vi "OceanOpticsInitialize.vi"(8 "error in (no error)":errorcluster, 11 "Numeric":i32) -> (0 "error out":errorcluster, 1 "getName":string, 2 "getSerialNumber":string, 3 ".NET Refnum out":refnum<k24>)   [LabVIEW 2016]
uses:
  C:/Program Files (x86)/Ocean Optics/OmniDriver/OOI_HOME/NETOmniDriver-NET40.dll
  Program Files (x86)/Ocean Optics/OmniDriver/OOI_HOME/NETOmniDriver-NET40.dll
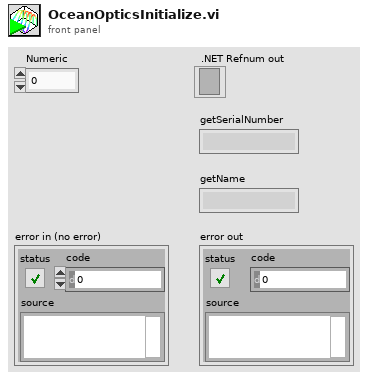
[diagram p1: front panel]
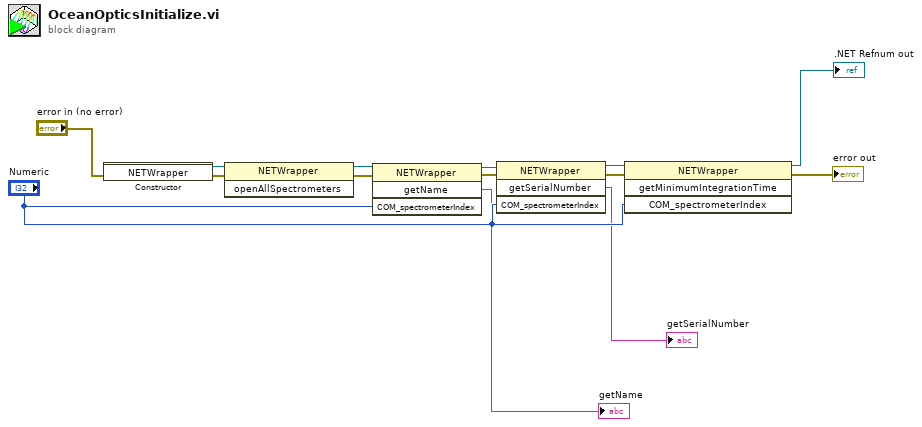
[diagram p0: block diagram]
diagram:
  n1 = constructor class="NETWrapper"(error in="error in (no error)") -> (reference out=w2:refnum<k24>, error out=w1:errorcluster)  [unwired: 2 in, 1 out]
  n2 = invoke class="NETWrapper" method="openAllSpectrometers"(reference=w2, error in=w1) -> (reference out=w8:refnum<k24>, error out=w7:errorcluster)  [unwired: 1 in, 1 out]
  n3 = invoke class="NETWrapper" method="getName"(reference=w8, error in=w7, "COM_spectrometerIndex"="Numeric") -> (reference out=w6:refnum<k24>, error out=w5:errorcluster, "getName"=→"getName":string)  [unwired: 1 in, 1 out]
  n4 = invoke class="NETWrapper" method="getSerialNumber"(reference=w6, error in=w5, "COM_spectrometerIndex"="Numeric") -> (reference out=w4:refnum<k24>, error out=w3:errorcluster, "getSerialNumber"=→"getSerialNumber":string)  [unwired: 1 in, 1 out]
  n5 = invoke class="NETWrapper" method="getMinimumIntegrationTime"(reference=w4, error in=w3, "COM_spectrometerIndex"="Numeric") -> (reference out=→".NET Refnum out":refnum<k24>, error out=→"error out":errorcluster)  [unwired: 1 in, 2 out]
